vi "PH_Beamline.color PA ED BL.vi"(0 "i ref in":refnum<vi>, 2 "Color State PA Exit to ED":i32, 5 "error in (no error)":errorcluster) -> (14 "i ref out":refnum<vi>, 19 "error out":errorcluster)   [LabVIEW 2014, in "PH_Beamline.lvlib"]
doc: "This Vi colors the PreAmp exit diagnose beamline elements."
uses:
  PH_Beamline.lvlib
  PH_Common/PH_Common.lvlib
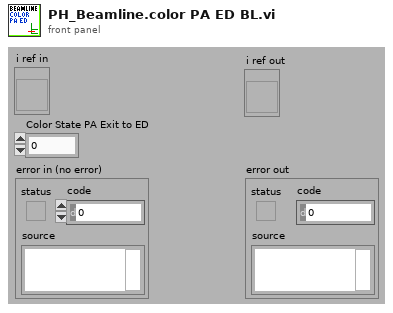
[diagram p1: front panel]
types:
  T1 = typedef "PH_Beamline.lvlib/PH_Beamline.i attribute.ctl" = cluster{"GUI Refs":cluster{"PA ok":refnum<vi>, "MA ok":refnum<vi>, "fs FE ok":refnum<vi>, "ns FE ok":refnum<vi>, "PA ED ok":refnum<vi>, "MAS ok":refnum<vi>, "Booster ok":refnum<vi>, "Mirrortower ok":refnum<vi>, "In.-Box ok":refnum<vi>, "Compressor ok":refnum<vi>, "Experiment LB ok":refnum<vi>, "Experiment LL ok":refnum<vi>, "PHELIX_Beckhoff_Watchdog":refnum<vi>, "Shutters closed":refnum<vi>, "uOPA ok":refnum<vi>, "Vacuum no shotcond Comp LB":refnum<vi>}, "Refs BL MA":refnum<vi>[], "Refs BL MA-IB":refnum<vi>[], "Refs BL fs":refnum<vi>[], "Refs BL PA ED":refnum<vi>[], "Refs BL MAS":refnum<vi>[], "Refs BL Boo":refnum<vi>[], "Refs BL ns":refnum<vi>[], "Refs BL Mirrortower":refnum<vi>[], "Refs BL Compressor":refnum<vi>[], "Refs BL Exp LB":refnum<vi>[], "Radiation Safety":cluster{"Exp Laserbay":cluster{"Ref Op Mode":refnum<vi>, "Ref Laserbay evacuated":refnum<vi>, "Tagname LB evacuated":string, "Shot Mode":T2, "Laserbay evacuated?":i32, "Tagname HV room locked":string, "HV room locked?":i32, "Ref HV room locked":refnum<vi>, "Tagname bridged?":string, "Ref Bridge":refnum<vi>, "I<1E18W/cm²":bool}, "Exp Laserlab":cluster{"Ref Op Mode":refnum<vi>, "Ref Laserlab evacuated":refnum<vi>, "Tagname LL evacuated":string, "Shot Mode":T2, "Laserlab evacuated?":i32, "Tagname bridged?":string, "Ref Bridge":refnum<vi>, "I<1E18W/cm²":bool}}, "Refs BL LL":refnum<vi>[], "PP Igni Heating GUI Refs":refnum<vi>[], "PP Igni Heating Tagnames ":string[], "Refs BL PA":cluster{"undelayed Line before Shutter":refnum<vi>[], "undelayed Line after Shutter":refnum<vi>[], "before Bypass":refnum<vi>[], "delayed Line before Shutter":refnum<vi>[], "delayed Line after Shutter":refnum<vi>[], "before Shutter Input":refnum<vi>[], "after Shutter Input":refnum<vi>[], "Bypass":refnum<vi>[], "before Shutter Exit":refnum<vi>[], "after Shutter Exit":refnum<vi>[], "to MA":refnum<vi>[], "to Lab":refnum<vi>[]}, "BL":cluster{"YLF_BL_Status":i32, "fs_BL_Status":i32, "fs_YLF_BL_Status":i32, "ns_BL_Status":i32, "PA_Input_BL_Status":i32, "PA_UnDelay_BL_Status":i32, "PA_Delay_BL_Status":i32, "PA_BL_Status":i32, "PA_Bypass_BL_Status":i32, "PA_Exit_BL_Status":i32, "PA_LL_BL_Status":i32, "LL_BL_Status":i32, "PA_MA_BL_Status":i32, "MA_Exit_BL_Status":i32, "MA_Z6_BL_Status":i32, "Z6_BL_Status":i32, "MA_LB_BL_Status":i32, "LB_TB2_BL_Status":i32, "PA_before_Bypass_BL_Status":i32, "LB_TB3_BL_Status":i32}, "State Subsystems":cluster{"PA":bool, "MA":bool, "ns FE":bool, "fs FE":bool, "PA ED":bool, "In.-Box":bool, "MAS":bool, "Booster":bool, "Mirrortower":bool, "Compressor":bool, "Experiment LB":bool, "Experiment LL":bool, "uOPA":bool}, "Status Subscriber Information":T3, "Refs BL uOPA":refnum<vi>[], "PA_Input_2_Beam_6PWpGUI not linked?":bool, "PA_Input_Delay_6PGUI not linked?":bool, "Settings":T6}
  T2 = typedef "PH_Beamline.lvlib/PH_Beamline.Operation Mode.ctl" = i32
  T3 = typedef "PH_Beamline.lvlib/PH_Beamline.Status Subscriber Information.ctl" = cluster{"fs Swich YLF":T4, "fs Exit Shutter":T4, "ns Exit Shutter":T4, "PA Input Shutter":T4, "PA PC WP":T4, "PA PC WP 2":T4, "PA Bypass In":T4, "PA Bypass Out":T4, "PA CH 1":T4, "PA delayed":T4, "PA non delayed":T4, "PA Exit Shutter":T4, "PA Switch Lab":T4, "PA Bridge CH Input MA":T4, "MA Diffusor IB":T4, "MA IB Ready":T4, "MA CH 1":T4, "MA CH 2":T4, "MA CH 3":T4, "MA CH 4":T4, "MA Shutter Align Cam":T4, "MA Position MM5":T4, "Calorimeter Switch":T4, "BL Z6 CH 9":T4, "BL Z6 Beamdump":T4, "BL Z6 Shutter":T4, "COS Sensitivity Switch":T4, "Exp LB Shutter":T4, "Exp LB TB 2":T4, "Exp LB TB 3":T4, "PA LL Input CH":T4, "PA LL Output CH":T4, "LL Comp Input Shutter":T4, "LL Comp Output Shutter":T4, "LL Comp FF Shutter":T4, "Exp LL Shutter":T4, "MA IM In IB":T4, "MA IM Out IB":T4, "MA DB In IB":T4, "MA DB Out IB":T4, "Exp LB Shutter Interlock":T4, "Exp LL Shutter Interlock":T4, "MM1 Force Sensor":T4}
  T4 = typedef "PH_BL-Master.lvlib/PH_BL-Master.Status Subscriber Information.ctl" = cluster{"Index of element":i32, "Attributeset":T5}
  T5 = typedef "PH_BL-Master.lvlib/PH_BL-Master.Attribute Set.ctl" = enum16{"Boolean Status Service Subscriber", "Picture Status Service Subscriber"}
  T6 = typedef "PH_Beamline_Chief.lvlib/PH_Beamline_Chief.Settings.ctl" = cluster{"PA Doublepass Mode":bool, "Compressor Vaccuum LB not relevant":bool, "Windowshutter TB2 not relevant":bool, "Windowshutter TB3 not relevant":bool}
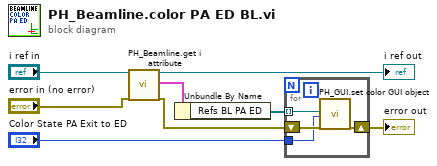
[diagram p0: block diagram]
diagram:
  n1 = call "PH_Beamline.get i attribute.vi"("i ref in"="i ref in", "error in (no error)"="error in (no error)") -> ("i ref out"=→"i ref out":refnum<vi>, "i attribute"=w8:T1, "error out"=w4:errorcluster)  [unwired: 15 in]
  n2 = Unbundle By Name(w8) -> ("Refs BL PA ED"=w6:refnum<vi>[])
  n3 = for "PA ED" {
    tunnel: w6 -> [w12] mode=indexing
    shift-right: [w10] -> w7
    shift-left: w4 -> [w11]
    tunnel: "Color State PA Exit to ED" -> [w9]
    n4 = call "PH_GUI.set color GUI object.vi"("GUI object Ref"=w12, "State"=w9, "error in (no error)"=w11) -> ("error out"=w10:errorcluster)  [unwired: 16 in]
  }
  "error out" <- w7
